vi "Main.vi"() -> ()   [LabVIEW 2013]
panel:
  in  "Divide 2":bool
  in  "Multiply 2":bool
  in  "Subtract 2":bool
  in  "Add 2":bool
  in  "Divide":bool
  in  "Stop":bool
  in  "Equal to":bool
  in  "Multiply":bool
  in  "Subtract":bool
  in  "Add":bool
  out "Display":string
  in  "Clear":bool
  in  "Nine":bool
  in  "Zero":bool
  in  "Delete":bool
  in  "Eight":bool
  in  "Seven":bool
  in  "Six":bool
  in  "Three":bool
  in  "Five":bool
  in  "Four":bool
  in  "Two":bool
  in  "One":bool
  # "KASIO"
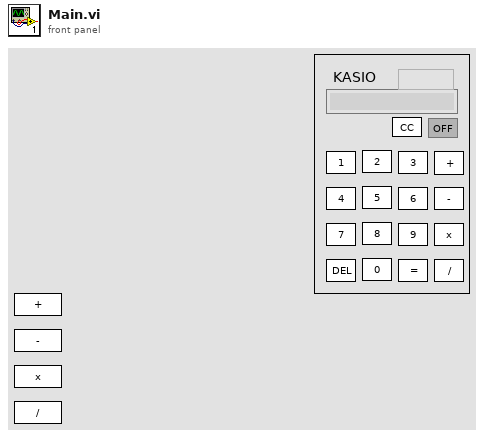
[diagram p1: front panel]
types:
  T1 = cluster{"Display":string, "First number":dbl, "operation":i32}
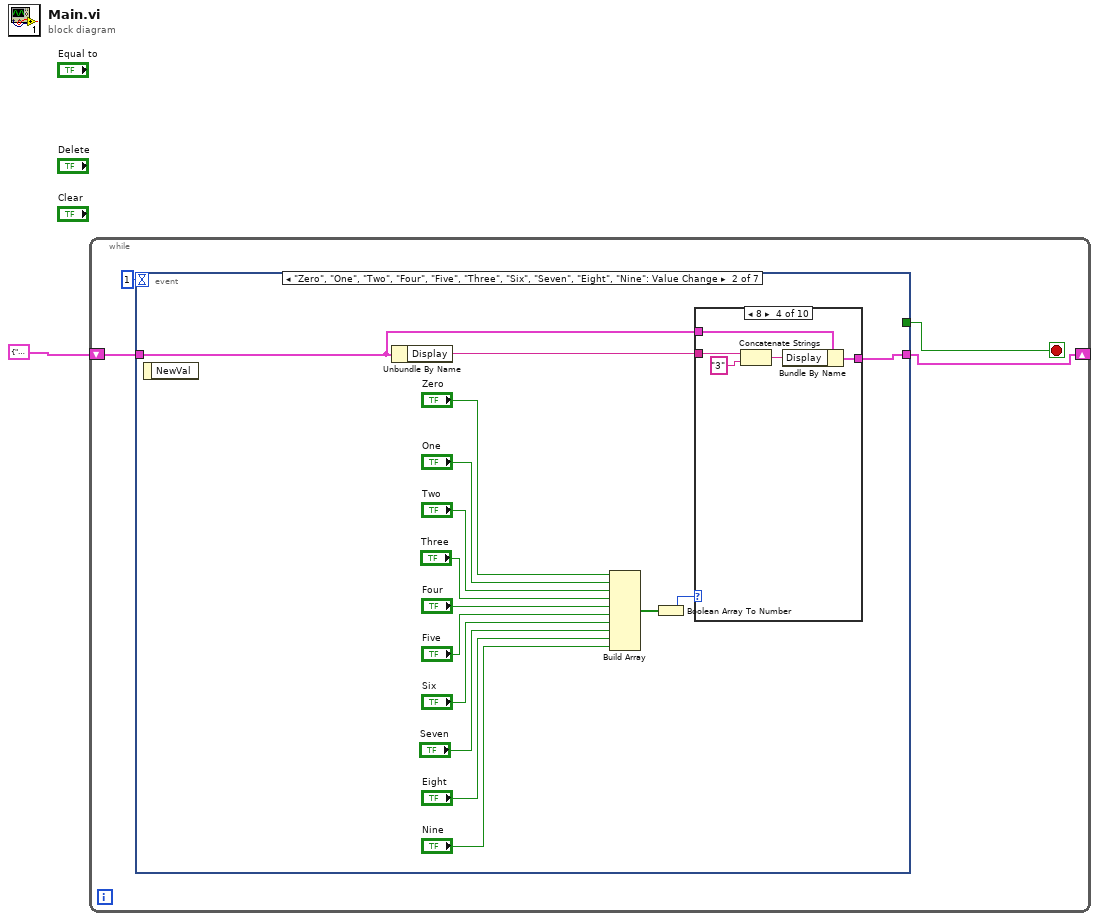
[diagram p0: block diagram]
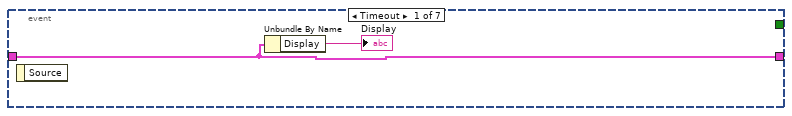
[diagram p2: hidden frame]
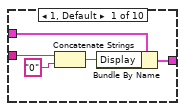
[diagram p3: hidden frame]
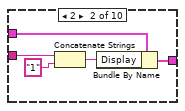
[diagram p4: hidden frame]
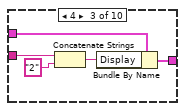
[diagram p5: hidden frame]
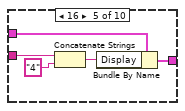
[diagram p6: hidden frame]
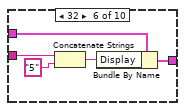
[diagram p7: hidden frame]
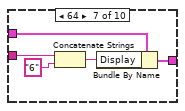
[diagram p8: hidden frame]
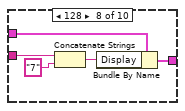
[diagram p9: hidden frame]
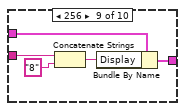
[diagram p10: hidden frame]
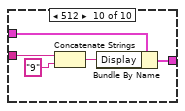
[diagram p11: hidden frame]
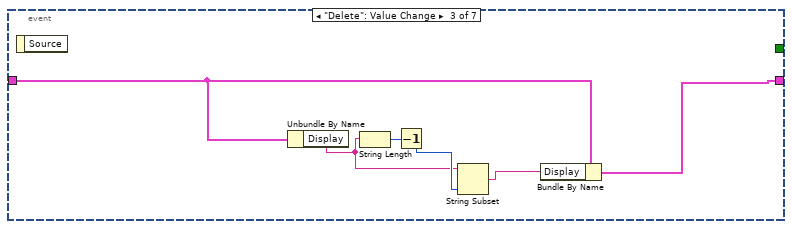
[diagram p12: hidden frame]
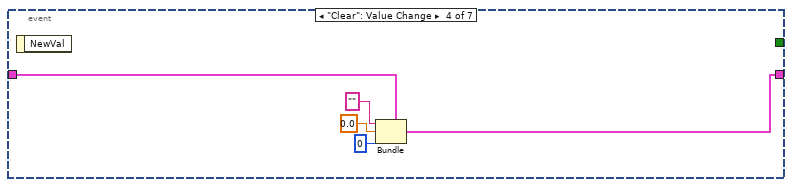
[diagram p13: hidden frame]
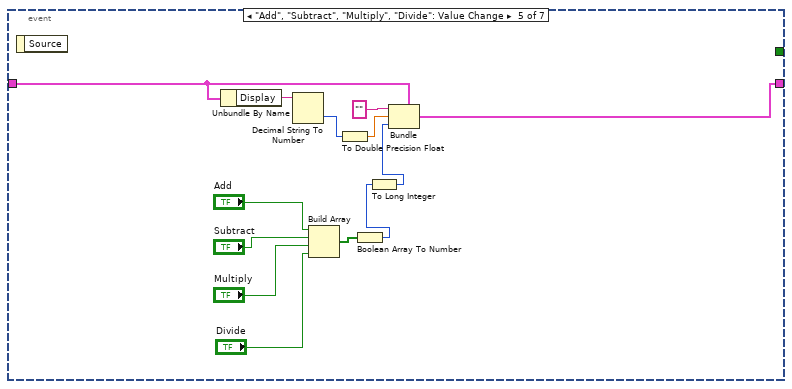
[diagram p14: hidden frame]
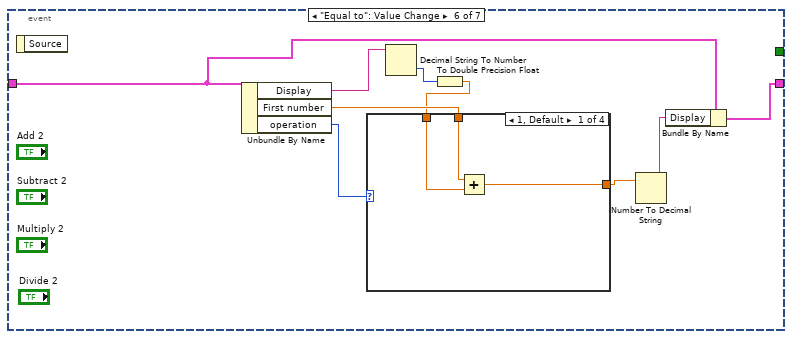
[diagram p15: hidden frame]
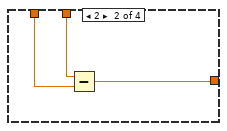
[diagram p16: hidden frame]
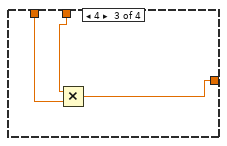
[diagram p17: hidden frame]
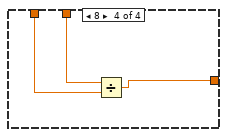
[diagram p18: hidden frame]
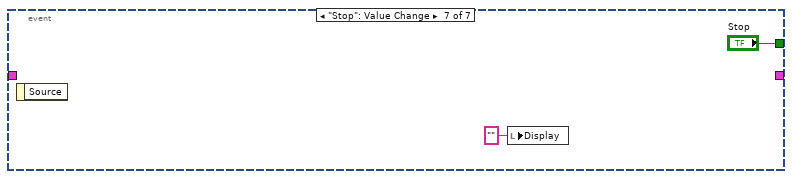
[diagram p19: hidden frame]
diagram:
  n1 = while {
    shift-right: [w2] -> _
    shift-left: T1 {"Display"="", "First number"=0.0, "operation"=0} -> [w5]
    stop <- w4 stop-if-true
    n2 = event shown="[1] \"Zero\", \"One\", \"Two\", \"Four\", \"Five\", \"Three\", \"Six\", \"Seven\", \"Eight\", \"Nine\": Value Change" {
      selector: _ -> [_ _ _ _ _ _ _]
      dyn-events: _ -> [_ _ _ _ _ _ _]
      timeout: 1 -> [_ _ _ _ _ _ _]
      tunnel: w5 -> [w6 w9 w75 w83 w95 w102 _]
      tunnel: [w6 w8 w74 w81 w94 w97 _] -> w2
      tunnel: [_ _ _ _ _ _ "Stop"] -> w4
      event Timeout {
        n3 = event-data() -> ()  [unwired: 1 in, 1 out]
        n4 = Unbundle By Name(w6) -> ("Display"=→"Display":string)
      }
      event "Zero", "One", "Two", "Four", "Five", "Three", "Six", "Seven", "Eight", "Nine": Value Change {
        n5 = event-data() -> ()  [unwired: 1 in, 1 out]
        n6 = Unbundle By Name(w9) -> ("Display"=w10:string)
        n7 = Build Array("Zero", "One", "Two", "Three", "Four", "Five", "Six", "Seven", "Eight", "Nine") -> (w12:bool[])
        n8 = Boolean Array To Number(Boolean array=w12) -> (number=w11:u32)
        n9 = case shown="8" w11 {
          tunnel: w10 -> [w26 w30 w35 w42 w45 w50 w55 w61 w65 w71]
          tunnel: w9 -> [w25 w31 w36 w41 w46 w51 w56 w60 w66 w69]
          tunnel: [w24 w29 w34 w40 w44 w49 w54 w59 w64 w70] -> w8
          frame 1, Default {
            n10 = Concatenate Strings(w26, "0" ("Display")) -> (w23:string)
            n11 = Bundle By Name(cluster=w25, "Display"=w23) -> (w24:T1)
          }
          frame 2 {
            n12 = Concatenate Strings(w30, "1" ("Display")) -> (w28:string)
            n13 = Bundle By Name(cluster=w31, "Display"=w28) -> (w29:T1)
          }
          frame 4 {
            n14 = Concatenate Strings(w35, "2" ("Display")) -> (w33:string)
            n15 = Bundle By Name(cluster=w36, "Display"=w33) -> (w34:T1)
          }
          frame 8 {
            n16 = Concatenate Strings(w42, "3" ("Display")) -> (w38:string)
            n17 = Bundle By Name(cluster=w41, "Display"=w38) -> (w40:T1)
          }
          frame 16 {
            n18 = Concatenate Strings(w45, "4" ("Display")) -> (w43:string)
            n19 = Bundle By Name(cluster=w46, "Display"=w43) -> (w44:T1)
          }
          frame 32 {
            n20 = Concatenate Strings(w50, "5" ("Display")) -> (w48:string)
            n21 = Bundle By Name(cluster=w51, "Display"=w48) -> (w49:T1)
          }
          frame 64 {
            n22 = Concatenate Strings(w55, "6" ("Display")) -> (w53:string)
            n23 = Bundle By Name(cluster=w56, "Display"=w53) -> (w54:T1)
          }
          frame 128 {
            n24 = Concatenate Strings(w61, "7" ("Display")) -> (w58:string)
            n25 = Bundle By Name(cluster=w60, "Display"=w58) -> (w59:T1)
          }
          frame 256 {
            n26 = Concatenate Strings(w65, "8" ("Display")) -> (w63:string)
            n27 = Bundle By Name(cluster=w66, "Display"=w63) -> (w64:T1)
          }
          frame 512 {
            n28 = Concatenate Strings(w71, "9" ("Display")) -> (w68:string)
            n29 = Bundle By Name(cluster=w69, "Display"=w68) -> (w70:T1)
          }
        }
      }
      event "Delete": Value Change {
        n30 = event-data() -> ()  [unwired: 1 in, 1 out]
        n31 = Unbundle By Name(w75) -> ("Display"=w73:string)
        n32 = String Length(string=w73) -> (length=w78:i32)
        n33 = Decrement(x=w78) -> (x-1=w77:i32)
        n34 = String Subset(string=w73, length (rest)=w77) -> (substring=w76:string)  [unwired: 1 in]
        n35 = Bundle By Name(cluster=w75, "Display"=w76) -> (w74:T1)
      }
      event "Clear": Value Change {
        n36 = event-data() -> ()  [unwired: 1 in, 1 out]
        n37 = Bundle(cluster=w83, "Display"="", "First number"=0.0, "operation"=0) -> (w81:T1)
      }
      event "Add", "Subtract", "Multiply", "Divide": Value Change {
        n38 = event-data() -> ()  [unwired: 1 in, 1 out]
        n39 = Unbundle By Name(w95) -> ("Display"=w96:string)
        n40 = Decimal String To Number(string=w96) -> (number=w85:i32)  [unwired: 2 in, 1 out]
        n41 = Build Array("Add", "Subtract", "Multiply", "Divide") -> (w89:bool[])
        n42 = To Double Precision Float(number=w85) -> (double precision float=w84:dbl)
        n43 = Boolean Array To Number(Boolean array=w89) -> (number=w88:u32)
        n44 = To Long Integer(number=w88) -> (32bit integer=w87:i32)
        n45 = Bundle(cluster=w95, "Display"="", "First number"=w84, "operation"=w87) -> (w94:T1)
      }
      event "Equal to": Value Change {
        n46 = event-data() -> ()  [unwired: 1 in, 1 out]
        n47 = Unbundle By Name(w102) -> ("Display"=w105:string, "First number"=w103:dbl, "operation"=w104:i32)
        n48 = Decimal String To Number(string=w105) -> (number=w99:i32)  [unwired: 2 in, 1 out]
        n49 = To Double Precision Float(number=w99) -> (double precision float=w98:dbl)
        n50 = case shown="1, Default" w104 {
          tunnel: w103 -> [w108 w110 w114 w117]
          tunnel: w98 -> [w107 w111 w113 w116]
          tunnel: [w106 w109 w112 w115] -> w101
          frame 1, Default {
            n51 = Add(x=w108, y=w107) -> (x+y=w106:dbl)
          }
          frame 2 {
            n52 = Subtract(x=w110, y=w111) -> (x-y=w109:dbl)
          }
          frame 4 {
            n53 = Multiply(x=w114, y=w113) -> (x*y=w112:dbl)
          }
          frame 8 {
            n54 = Divide(x=w117, y=w116) -> (x/y=w115:dbl)
          }
        }
        n55 = Number To Decimal String(number=w101) -> (decimal integer string=w100:string)  [unwired: 1 in]
        n56 = Bundle By Name(cluster=w102, "Display"=w100) -> (w97:T1)
      }
      event "Stop": Value Change {
        n57 = event-data() -> ()  [unwired: 1 in, 1 out]
        n58 = local write "Display"("" ("Display")) -> ()
      }
    }
  }
